vi "Main Page.vi"(8 "error in (no error)":errorcluster, 11 "Node Ptr":T1 format="%.0x") -> (0 "error out":errorcluster)   [LabVIEW 2019, in "HLA Custom Device System Explorer.lvlib"]
uses:
  HLA Custom Device System Explorer.lvlib
  <vilib>/NI VeriStand/Custom Device API/Custom Device Item Ref.ctl
  <vilib>/NI VeriStand/Custom Device API/Get Item Property (U16).vi
  <vilib>/NI VeriStand/Custom Device API/Set Item Property (U16).vi
  Shared/Constants.vi
  <vilib>/NI VeriStand/Custom Device API/Set Item Property (String).vi
  <vilib>/NI VeriStand/Custom Device API/Set Item Property (Path).vi
  <vilib>/NI VeriStand/Custom Device API/Custom Device API.lvlib
  Shared/HLA Custom Device Shared.lvlib
panel:
  in  "custom FOM path on RT":string
  in  "MAK configuration file (.mtl)":path
  in  "FOM Module":path
  in  "Federate Type":string
  in  "Federation Execution Name":string
  in  "Local Designator Settings":string
  in  "Async Timeout (ms)":u16
  out "Version":string
  in  "SHDocVw.IWebBrowser":refnum<k7>(container)
  in  "Specific Header":cluster{"Section Name":string}={"Section Name"="Custom Device Item Settings"}
  in  "General Header":cluster{"Section Name":string}={"Section Name"="General Custom Device Settings"}
  in  "Description":string
  in  "Name":string
  # "keep this field empty if you want to use the \nMAK configuration file as local designator settings"
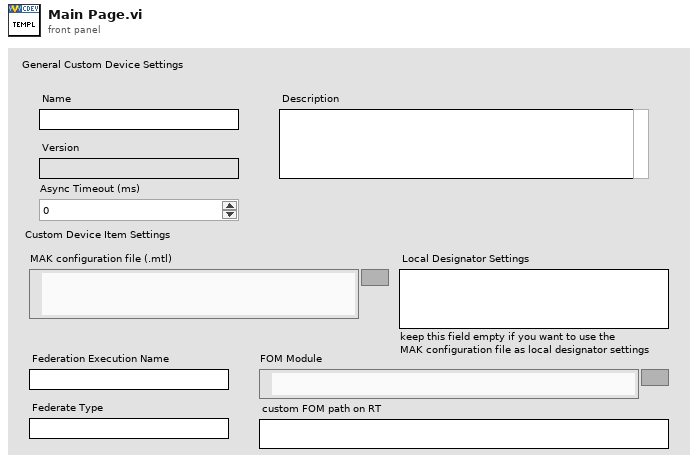
[diagram p1: front panel]
types:
  T1 = typedef "Custom Device API.lvlib/Custom Device Item Ref.ctl" = u64
  T2 = typedef "Custom Device API.lvlib/Custom Device Item Info.ctl" = cluster{"Name":string, "Is Channel":bool, "GUID":string, "Is Waveform":bool}
  T3 = typedef "HLA Custom Device Shared.lvlib/main_page_config.ctl" = cluster{"Federate Execution Name":string, "Federate Type":string, "Local Designator Settings":string, "FOM Module":path, "mak mtl file":path}
  T4 = typedef "Custom Device API.lvlib/Custom Device Commands.ctl" = enum16{"Default", "Item renamed", "Shutdown", "Dynamic button pressed"}
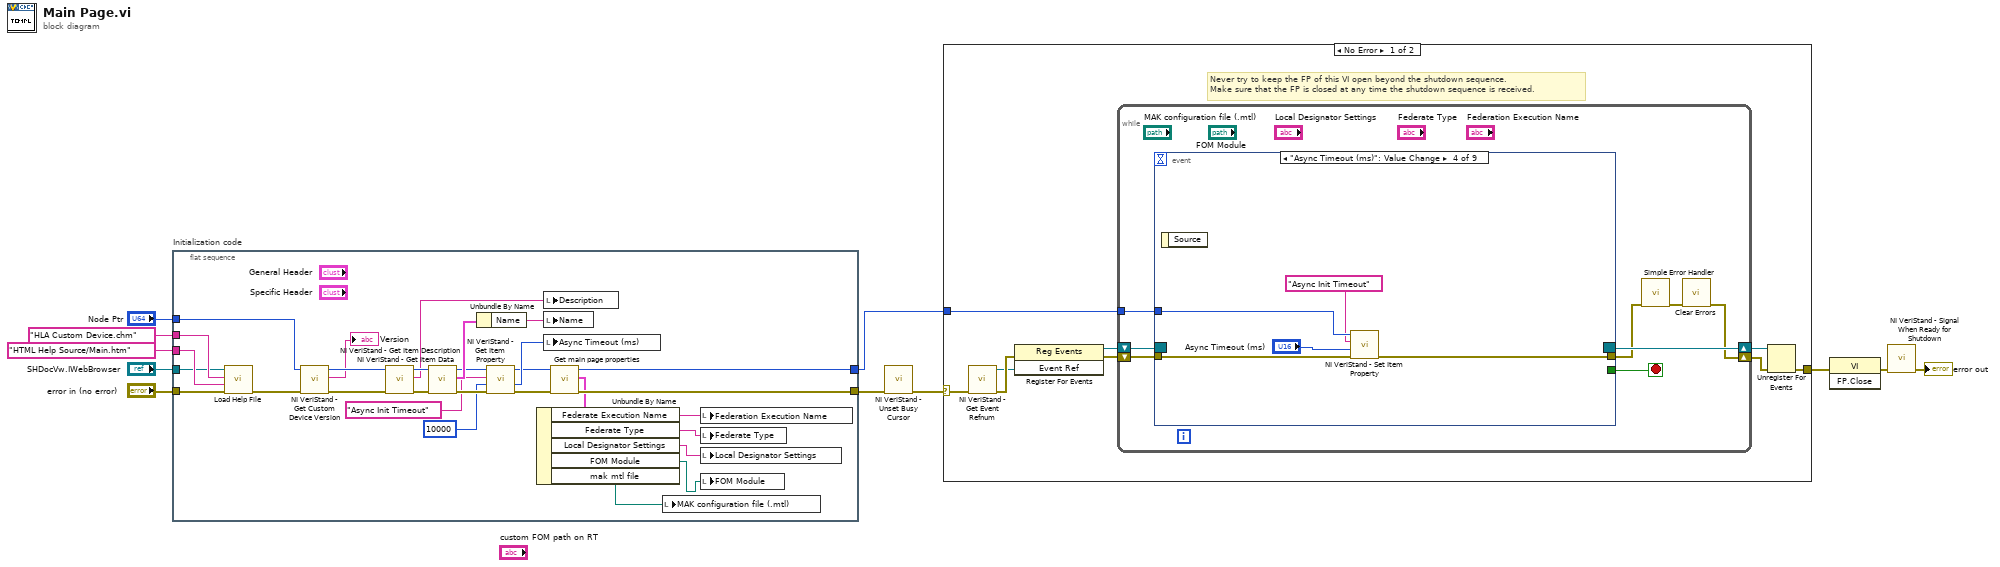
[diagram p0: block diagram]
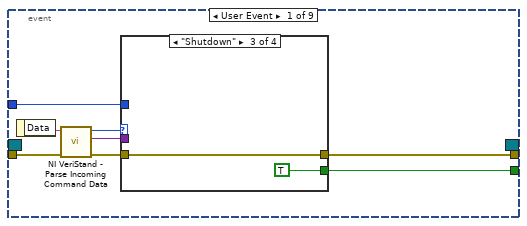
[diagram p2: hidden frame]
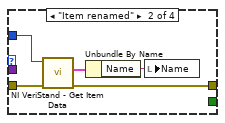
[diagram p4: hidden frame]
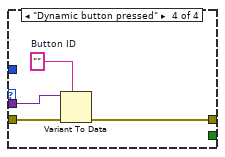
[diagram p5: hidden frame]
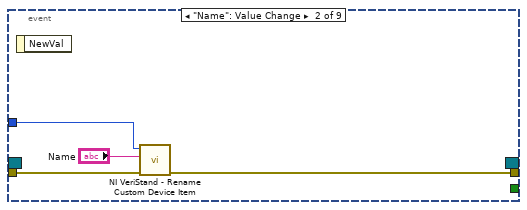
[diagram p6: hidden frame]
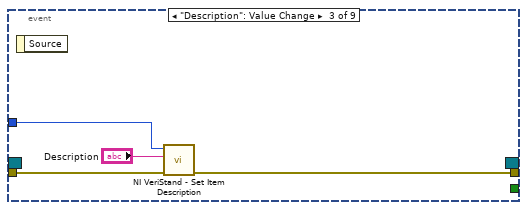
[diagram p7: hidden frame]
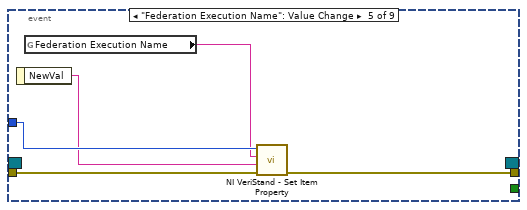
[diagram p8: hidden frame]
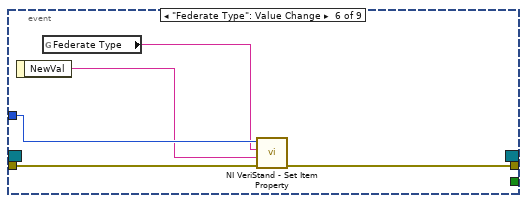
[diagram p9: hidden frame]
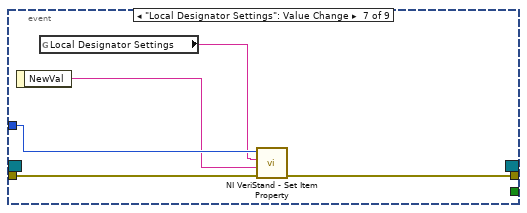
[diagram p10: hidden frame]
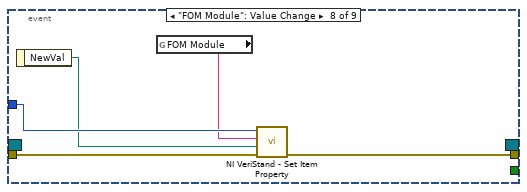
[diagram p11: hidden frame]
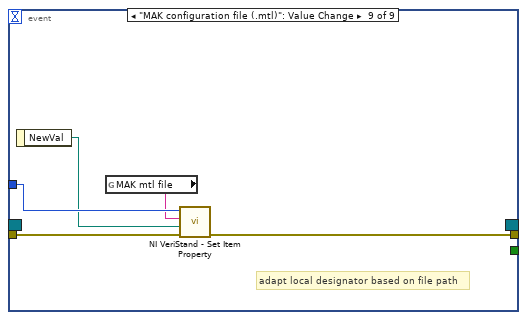
[diagram p12: hidden frame]
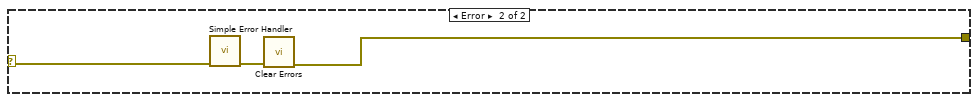
[diagram p13: hidden frame]
diagram:
  n1 = flat-sequence "Initialization code" {
    tunnel: "error in (no error)" -> [w31]
    tunnel: "Node Ptr" -> [w37]
    tunnel: [w19] -> w7
    tunnel: [w18] -> w4
    tunnel: "SHDocVw.IWebBrowser" -> [w27]
    tunnel: "HTML Help Source/Main.htm" ("HTML File") -> [w28]
    tunnel: "HLA Custom Device.chm" ("CD_CHM_FileName") -> [w29]
    frame #0 {
      n2 = call "Load Help File.vi"("error in (no error)"=w31, "HTML File to Load"=w28, "Main CHM File"=w29, "Browser"=w27) -> ("error out"=w30:errorcluster)  [unwired: 7 in]
      n3 = call <vilib>:"NI VeriStand - Get Custom Device Version.vi"("error in (no error)"=w30, "Device Ref in"=w37) -> ("error out"=w36:errorcluster, "Value"=→"Version":string, "Device Ref out"=w35:T1)  [unwired: 7 in]
      n4 = call <vilib>:"NI VeriStand - Get Item Description.vi"("error in (no error)"=w36, "Item Ref in"=w35) -> ("error out"=w39:errorcluster, "Description"=w32:string, "Item Ref out"=w40:T1)  [unwired: 7 out]
      n5 = call <vilib>:"NI VeriStand - Get Item Data.vi"("error in (no error)"=w39, "Item Ref in"=w40) -> ("error out"=w26:errorcluster, "Item Info"=w38:T2, "Item Ref out"=w25:T1)  [unwired: 7 out]
      n6 = Unbundle By Name(w38) -> ("Name"=w33:string)
      n7 = call-poly <vilib>:"NI VeriStand - Get Item Property.vi"("error in (no error)"=w26, "Default Value"=u16 10000, "Property Name"="Async Init Timeout", "Item Ref in"=w25) -> ("error out"=w20:errorcluster, "Value"=w24:u16, "Item Ref out"=w21:T1)  [unwired: 4 in, 1 out]
      n8 = local write "Description"(w32) -> ()
      n9 = local write "Name"(w33) -> ()
      n10 = local write "Async Timeout (ms)"(w24) -> ()
      n11 = call "Get main page properties.vi"("error in"=w20, "Item Ref in"=w21) -> ("error out"=w19:errorcluster, "main page properties"=w17:T3, "Item Ref out"=w18:T1)  [unwired: 7 in]
      n12 = Unbundle By Name(w17) -> ("Federate Execution Name"=w16:string, "Federate Type"=w15:string, "Local Designator Settings"=w14:string, "FOM Module"=w13:path, "mak mtl file"=w12:path)
      n13 = local write "MAK configuration file (.mtl)"(w12) -> ()
      n14 = local write "Federation Execution Name"(w16) -> ()
      n15 = local write "Federate Type"(w15) -> ()
      n16 = local write "Local Designator Settings"(w14) -> ()
      n17 = local write "FOM Module"(w13) -> ()
    }
  }
  n18 = call <vilib>:"NI VeriStand - Unset Busy Cursor.vi"("error in (no error)"=w7) -> ("error out"=w6:errorcluster)  [unwired: 10 out]
  n19 = case shown="No Error" w6 {
    selector: w6 -> [w41 w118]
    tunnel: [w46 w116] -> w11
    tunnel: w4 -> [w42 _]
    frame No Error {
      # "Never try to keep the FP of this VI open beyond the shutdown sequence.\nMake sure that the FP is closed at any time the shutdown sequence is received."
      n20 = call <vilib>:"NI VeriStand - Get Event Refnum.vi"("error in (no error)"=w41) -> ("error out"=w49:errorcluster, "Event Ref"=w45:refnum<user-event>)  [unwired: 9 out]
      n21 = register-events(error in=w49, w45) -> (reference out=w43:refnum<event-registration>, error out=w44:errorcluster)  [unwired: 1 in]
      n22 = while {
        tunnel: w42 -> [w53]
        shift-right: [w50] -> w47
        shift-left: w44 -> [w56]
        shift-right: [w57] -> w48
        shift-left: w43 -> [w55]
        stop <- w54 stop-if-true
        n23 = event shown="[3] \"Async Timeout (ms)\": Value Change" {
          selector: w55 -> [_ _ _ _ _ _ _ _ _]
          dyn-events: [_ _ _ _ _ _ _ _ _] -> w57
          timeout: _ -> [_ _ _ _ _ _ _ _ _]
          tunnel: w56 -> [w65 w81 w84 w90 w95 w100 w105 w110 w115]
          tunnel: [w61 _ _ _ _ _ _ _ _] -> w54
          tunnel: [w60 w80 w83 w87 w94 w99 w104 w109 w111] -> w52
          tunnel: w53 -> [w59 w79 w85 w89 w93 w98 w103 w108 w114]
          event User Event {
            n24 = event-data() -> ("Data"=w64:string)  [unwired: 1 out]
            n25 = call <vilib>:"NI VeriStand - Parse Incoming Command Data.vi"("error in (no error)"=w65, "Incoming data"=w64) -> ("error out"=w63:errorcluster, "Outgoing data"=w58:variant, "Action"=w62:T4)  [unwired: 7 out]
            n26 = case shown="\"Shutdown\"" w62 {
              tunnel: w63 -> [w66 w71 w72 w77]
              tunnel: [_ _ TRUE _] -> w61
              tunnel: [w66 w68 w72 w74] -> w60
              tunnel: w59 -> [_ w70 _ _]
              tunnel: w58 -> [_ _ _ w76]
              frame "Default", Default {
              }
              frame "Item renamed" {
                n27 = call <vilib>:"NI VeriStand - Get Item Data.vi"("error in (no error)"=w71, "Item Ref in"=w70) -> ("error out"=w68:errorcluster, "Item Info"=w69:T2)  [unwired: 8 out]
                n28 = Unbundle By Name(w69) -> ("Name"=w67:string)
                n29 = local write "Name"(w67) -> ()
              }
              frame "Shutdown" {
              }
              frame "Dynamic button pressed" {
                w75 = ""  # Button ID
                n30 = Variant To Data(error in=w77, type=w75, Variant=w76) -> (error out=w74:errorcluster)  [unwired: 1 out]
              }
            }
          }
          event "Name": Value Change {
            n31 = event-data() -> ()  [unwired: 2 out]
            n32 = call <vilib>:"NI VeriStand - Rename Custom Device Item.vi"("error in (no error)"=w81, "New Name"="Name", "Item Ref in"=w79) -> ("error out"=w80:errorcluster)  [unwired: 1 in, 7 out]
          }
          event "Description": Value Change {
            n33 = event-data() -> ()  [unwired: 2 out]
            n34 = call <vilib>:"NI VeriStand - Set Item Description.vi"("error in (no error)"=w84, "Description"="Description", "Item Ref in"=w85) -> ("error out"=w83:errorcluster)  [unwired: 8 out]
          }
          event "Async Timeout (ms)": Value Change {
            n35 = event-data() -> ()  [unwired: 2 out]
            n36 = call-poly <vilib>:"NI VeriStand - Set Item Property.vi"("error in (no error)"=w90, "Value"="Async Timeout (ms)", "Property Name"="Async Init Timeout", "Item Ref in"=w89) -> ("error out"=w87:errorcluster)  [unwired: 5 in, 2 out]
          }
          event "Federation Execution Name": Value Change {
            n37 = event-data() -> ("NewVal"=w91:string)  [unwired: 1 out]
            n38 = global read "Constants.vi" "Federation Execution Name"() -> (w92:string)
            n39 = call-poly <vilib>:"NI VeriStand - Set Item Property.vi"("error in (no error)"=w95, "Value"=w91, "Property Name"=w92, "Item Ref in"=w93) -> ("error out"=w94:errorcluster)  [unwired: 5 in, 2 out]
          }
          event "Federate Type": Value Change {
            n40 = event-data() -> ("NewVal"=w96:string)  [unwired: 1 out]
            n41 = global read "Constants.vi" "Federate Type"() -> (w97:string)
            n42 = call-poly <vilib>:"NI VeriStand - Set Item Property.vi"("error in (no error)"=w100, "Value"=w96, "Property Name"=w97, "Item Ref in"=w98) -> ("error out"=w99:errorcluster)  [unwired: 5 in, 2 out]
          }
          event "Local Designator Settings": Value Change {
            n43 = event-data() -> ("NewVal"=w101:string)  [unwired: 1 out]
            n44 = global read "Constants.vi" "Local Designator Settings"() -> (w102:string)
            n45 = call-poly <vilib>:"NI VeriStand - Set Item Property.vi"("error in (no error)"=w105, "Value"=w101, "Property Name"=w102, "Item Ref in"=w103) -> ("error out"=w104:errorcluster)  [unwired: 5 in, 2 out]
          }
          event "FOM Module": Value Change {
            n46 = event-data() -> ("NewVal"=w106:path)  [unwired: 1 out]
            n47 = global read "Constants.vi" "FOM Module"() -> (w107:string)
            n48 = call-poly <vilib>:"NI VeriStand - Set Item Property.vi"("error in (no error)"=w110, "Value"=w106, "Property Name"=w107, "Item Ref in"=w108) -> ("error out"=w109:errorcluster)  [unwired: 5 in, 2 out]
          }
          event "MAK configuration file (.mtl)": Value Change {
            # "adapt local designator based on file path"
            n49 = event-data() -> ("NewVal"=w112:path)  [unwired: 1 out]
            n50 = global read "Constants.vi" "MAK mtl file"() -> (w113:string)
            n51 = call-poly <vilib>:"NI VeriStand - Set Item Property.vi"("error in (no error)"=w115, "Value"=w112, "Property Name"=w113, "Item Ref in"=w114) -> ("error out"=w111:errorcluster)  [unwired: 5 in, 2 out]
          }
        }
        n52 = call <vilib>:"Simple Error Handler.vi"("error in (no error)"=w52) -> ("error out"=w51:errorcluster)  [unwired: 1 in, 7 out]
        n53 = call <vilib>:"Clear Errors.vi"("error in (no error)"=w51) -> ("error out"=w50:errorcluster)  [unwired: 1 in, 5 out]
      }
      n54 = Unregister For Events(event registration refnum=w48, error in=w47) -> (error out=w46:errorcluster)
    }
    frame Error {
      n55 = call <vilib>:"Simple Error Handler.vi"("error in (no error)"=w118) -> ("error out"=w117:errorcluster)  [unwired: 1 in, 7 out]
      n56 = call <vilib>:"Clear Errors.vi"("error in (no error)"=w117) -> ("error out"=w116:errorcluster)  [unwired: 1 in, 5 out]
    }
  }
  n57 = invoke class="VI" method="FP.Close"(error in=w11) -> (error out=w10:errorcluster)  [unwired: 2 in, 2 out]
  n58 = call <vilib>:"NI VeriStand - Signal When Ready for Shutdown.vi"("error in (no error)"=w10) -> ("error out"=→"error out":errorcluster)  [unwired: 10 out]
